vi "Process Live Data Q EMG.vi"(8 "error in (no error)":errorcluster, 10 "Live Data Q Elements":cluster{"NI Data Waveforms":waveform(dbl)[]}[](array[cluster]), 11 "NI Force Task in":refnum<class "NI Force Task.lvclass">) -> (0 "error out":errorcluster, 3 "NI Force Task out":refnum<class "NI Force Task.lvclass">)   [LabVIEW 2020, in "NI Force Task.lvlib" / "NI Force Task.lvclass"]
uses:
  NI Force Task.lvclass
  NI Force Task.lvclass/NI Force Task.ctl
  <vilib>/Analysis/baseanly.llb/Mean (DBL).vi
  <vilib>/Analysis/NI_AALBase.lvlib
  Task Viewer Messages/Receive Q Msg/Receive Q Msg.lvclass
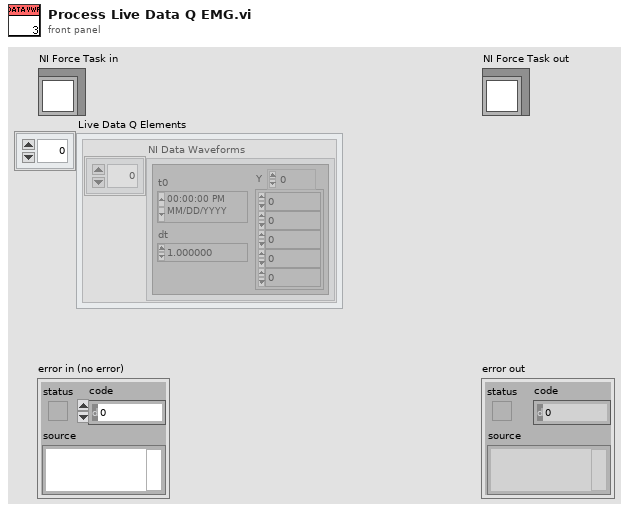
[diagram p1: front panel]
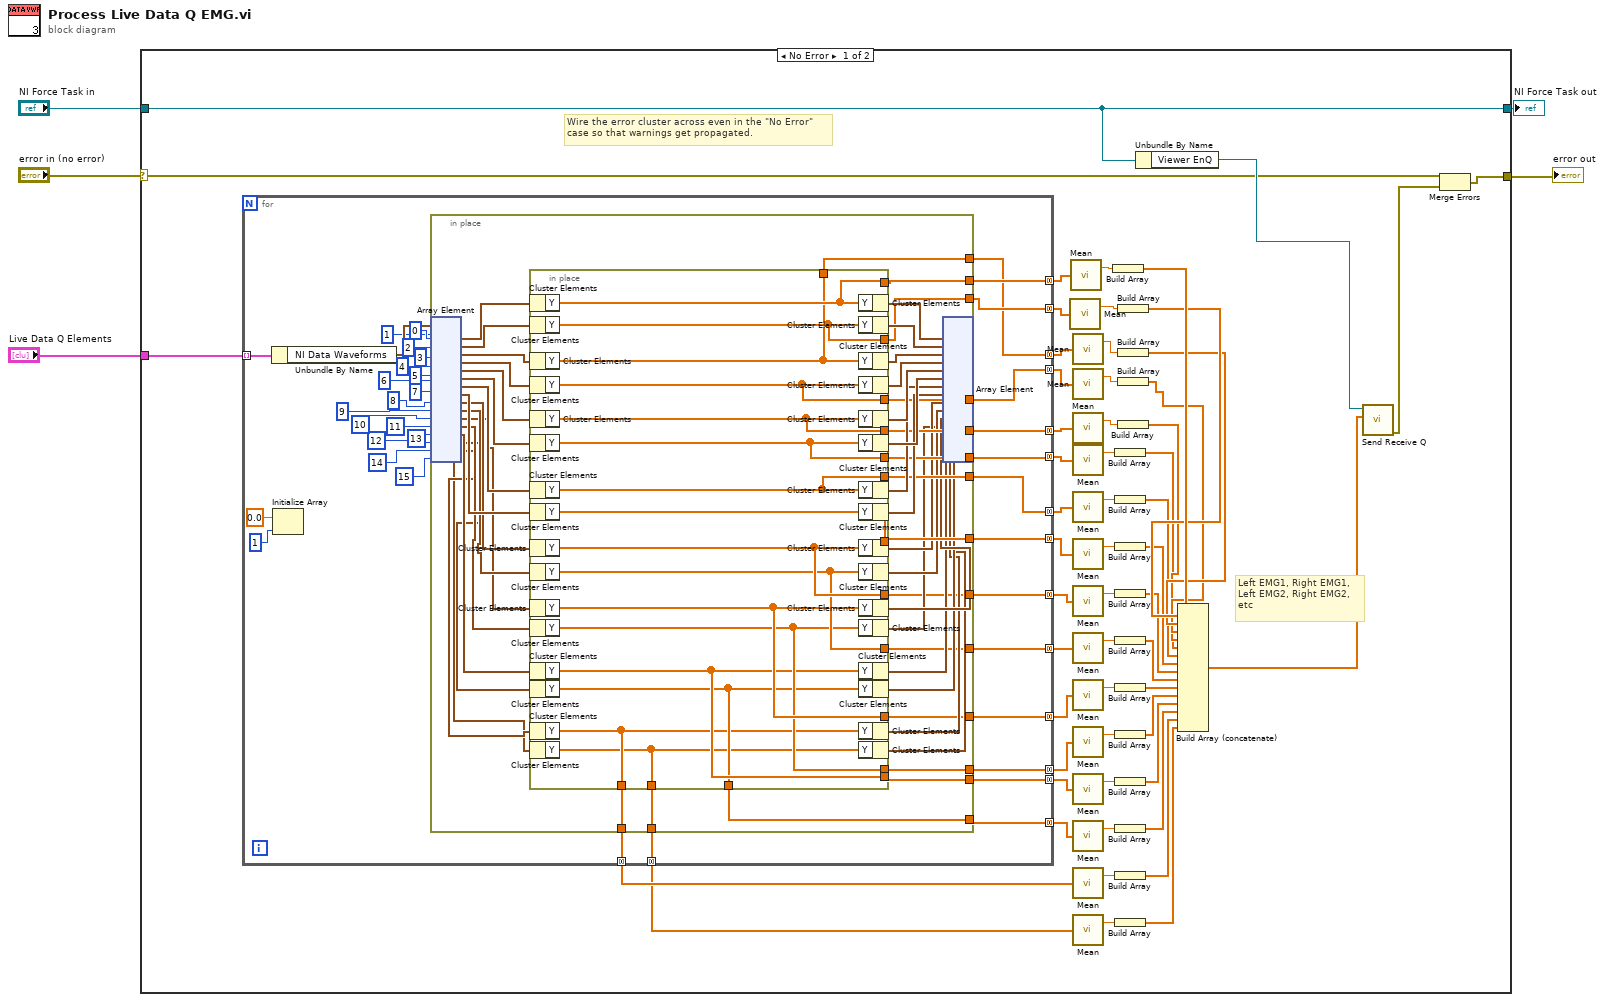
[diagram p0: block diagram]
diagram:
  n1 = case shown="No Error" "error in (no error)" {
    selector: "error in (no error)" -> [w53 w161]
    tunnel: [w60 w162] -> w3
    tunnel: "NI Force Task in" -> [w60 w162]
    tunnel: "Live Data Q Elements" -> [w59 _]
    tunnel: [w57 w161] -> w1
    frame No Error {
      # "Left EMG1, Right EMG1,\nLeft EMG2, Right EMG2,\netc"
      # "Wire the error cluster across even in the \"No Error\"\ncase so that warnings get propagated."
      n2 = for {
        tunnel: w59 -> [w96] mode=indexing
        tunnel: [w84] -> w52 mode=concatenating
        tunnel: [w83] -> w51 mode=concatenating
        tunnel: [w82] -> w48 mode=concatenating
        tunnel: [w81] -> w50 mode=concatenating
        tunnel: [w80] -> w49 mode=concatenating
        tunnel: [w79] -> w47 mode=concatenating
        tunnel: [w78] -> w46 mode=concatenating
        tunnel: [w77] -> w45 mode=concatenating
        tunnel: [w68] -> w13 mode=concatenating
        tunnel: [w67] -> w12 mode=concatenating
        tunnel: [w66] -> w11 mode=concatenating
        tunnel: [w65] -> w10 mode=concatenating
        tunnel: [w64] -> w9 mode=concatenating
        tunnel: [w63] -> w8 mode=concatenating
        tunnel: [w62] -> w7 mode=concatenating
        tunnel: [w61] -> w6 mode=concatenating
        n3 = Unbundle By Name(w96) -> ("NI Data Waveforms"=w93:waveform(dbl)[])
        n4 = Initialize Array(0.0 ("element"), 1 ("dimension size")) -> ()  [unwired: 1 out]
        n5 = in-place {
          in-place-border: [w128] -> w84
          in-place-border: [w127] -> w83
          in-place-border: [w126] -> w82
          in-place-border: [w125] -> w81
          in-place-border: [w124] -> w80
          in-place-border: [w123] -> w79
          in-place-border: [w122] -> w78
          in-place-border: [w121] -> w77
          in-place-border: [w104] -> w68
          in-place-border: [w103] -> w67
          in-place-border: [w102] -> w66
          in-place-border: [w101] -> w65
          in-place-border: [w100] -> w64
          in-place-border: [w99] -> w63
          in-place-border: [w98] -> w62
          in-place-border: [w97] -> w61
          n6 = in-place-array #1(w93, 0, 1, 2, 3, 4, 5, 6, 7, 8, 9, 10, 11, 12, 13, 14, 15) -> (w144:waveform(dbl), w143:waveform(dbl), w142:waveform(dbl), w141:waveform(dbl), w140:waveform(dbl), w139:waveform(dbl), w138:waveform(dbl), w137:waveform(dbl), w120:waveform(dbl), w119:waveform(dbl), w118:waveform(dbl), w117:waveform(dbl), w116:waveform(dbl), w115:waveform(dbl), w114:waveform(dbl), w113:waveform(dbl))
          n7 = in-place {
            in-place-border: [w160] -> w128
            in-place-border: [w159] -> w127
            in-place-border: [w158] -> w126
            in-place-border: [w157] -> w125
            in-place-border: [w156] -> w124
            in-place-border: [w155] -> w123
            in-place-border: [w154] -> w122
            in-place-border: [w153] -> w121
            in-place-border: [w152] -> w104
            in-place-border: [w151] -> w103
            in-place-border: [w150] -> w102
            in-place-border: [w149] -> w101
            in-place-border: [w148] -> w100
            in-place-border: [w147] -> w99
            in-place-border: [w146] -> w98
            in-place-border: [w145] -> w97
            n8 = in-place-cluster #2(w144) -> ("Y"=w160:dbl[])
            n9 = in-place-cluster #3(w143) -> ("Y"=w159:dbl[])
            n10 = in-place-cluster #4(w142) -> ("Y"=w158:dbl[])
            n11 = in-place-cluster #5(w141) -> ("Y"=w157:dbl[])
            n12 = in-place-cluster #6(w140) -> ("Y"=w156:dbl[])
            n13 = in-place-cluster #7(w139) -> ("Y"=w155:dbl[])
            n14 = in-place-cluster #8(w138) -> ("Y"=w154:dbl[])
            n15 = in-place-cluster #9(w137) -> ("Y"=w153:dbl[])
            n16 = in-place-cluster #10(w120) -> ("Y"=w152:dbl[])
            n17 = in-place-cluster #11(w119) -> ("Y"=w151:dbl[])
            n18 = in-place-cluster #12(w118) -> ("Y"=w150:dbl[])
            n19 = in-place-cluster #13(w117) -> ("Y"=w149:dbl[])
            n20 = in-place-cluster #14(w116) -> ("Y"=w148:dbl[])
            n21 = in-place-cluster #15(w115) -> ("Y"=w147:dbl[])
            n22 = in-place-cluster #16(w114) -> ("Y"=w146:dbl[])
            n23 = in-place-cluster #17(w113) -> ("Y"=w145:dbl[])
            n24 = in-place-cluster #2("Y"=w160) -> (w136:waveform(dbl))
            n25 = in-place-cluster #3("Y"=w159) -> (w135:waveform(dbl))
            n26 = in-place-cluster #4("Y"=w158) -> (w134:waveform(dbl))
            n27 = in-place-cluster #5("Y"=w157) -> (w133:waveform(dbl))
            n28 = in-place-cluster #6("Y"=w156) -> (w132:waveform(dbl))
            n29 = in-place-cluster #7("Y"=w155) -> (w131:waveform(dbl))
            n30 = in-place-cluster #8("Y"=w154) -> (w130:waveform(dbl))
            n31 = in-place-cluster #9("Y"=w153) -> (w129:waveform(dbl))
            n32 = in-place-cluster #10("Y"=w152) -> (w112:waveform(dbl))
            n33 = in-place-cluster #11("Y"=w151) -> (w111:waveform(dbl))
            n34 = in-place-cluster #12("Y"=w150) -> (w110:waveform(dbl))
            n35 = in-place-cluster #13("Y"=w149) -> (w109:waveform(dbl))
            n36 = in-place-cluster #14("Y"=w148) -> (w108:waveform(dbl))
            n37 = in-place-cluster #15("Y"=w147) -> (w107:waveform(dbl))
            n38 = in-place-cluster #16("Y"=w146) -> (w106:waveform(dbl))
            n39 = in-place-cluster #17("Y"=w145) -> (w105:waveform(dbl))
          }
          n40 = in-place-array #1(w136, w135, w134, w133, w132, w131, w130, w129, w112, w111, w110, w109, w108, w107, w106, w105) -> ()  [unwired: 17 out]
        }
      }
      n41 = call-poly <vilib>:"Mean.vi"("X"=w51) -> ("mean"=w54:dbl)  [unwired: 1 out]
      n42 = call-poly <vilib>:"Mean.vi"("X"=w52) -> ("mean"=w55:dbl)  [unwired: 1 out]
      n43 = call-poly <vilib>:"Mean.vi"("X"=w48) -> ("mean"=w44:dbl)  [unwired: 1 out]
      n44 = call-poly <vilib>:"Mean.vi"("X"=w50) -> ("mean"=w43:dbl)  [unwired: 1 out]
      n45 = call-poly <vilib>:"Mean.vi"("X"=w49) -> ("mean"=w42:dbl)  [unwired: 1 out]
      n46 = call-poly <vilib>:"Mean.vi"("X"=w47) -> ("mean"=w41:dbl)  [unwired: 1 out]
      n47 = call-poly <vilib>:"Mean.vi"("X"=w46) -> ("mean"=w40:dbl)  [unwired: 1 out]
      n48 = call-poly <vilib>:"Mean.vi"("X"=w45) -> ("mean"=w39:dbl)  [unwired: 1 out]
      n49 = call-poly <vilib>:"Mean.vi"("X"=w13) -> ("mean"=w29:dbl)  [unwired: 1 out]
      n50 = call-poly <vilib>:"Mean.vi"("X"=w12) -> ("mean"=w28:dbl)  [unwired: 1 out]
      n51 = call-poly <vilib>:"Mean.vi"("X"=w11) -> ("mean"=w27:dbl)  [unwired: 1 out]
      n52 = call-poly <vilib>:"Mean.vi"("X"=w10) -> ("mean"=w26:dbl)  [unwired: 1 out]
      n53 = call-poly <vilib>:"Mean.vi"("X"=w9) -> ("mean"=w25:dbl)  [unwired: 1 out]
      n54 = call-poly <vilib>:"Mean.vi"("X"=w8) -> ("mean"=w24:dbl)  [unwired: 1 out]
      n55 = call-poly <vilib>:"Mean.vi"("X"=w7) -> ("mean"=w23:dbl)  [unwired: 1 out]
      n56 = call-poly <vilib>:"Mean.vi"("X"=w6) -> ("mean"=w22:dbl)  [unwired: 1 out]
      n57 = Build Array(w55) -> (w37:dbl[])
      n58 = Build Array(w41) -> (w32:dbl[])
      n59 = Build Array(w40) -> (w31:dbl[])
      n60 = Build Array(w39) -> (w30:dbl[])
      n61 = Build Array(w29) -> (w21:dbl[])
      n62 = Build Array(w28) -> (w20:dbl[])
      n63 = Build Array(w27) -> (w19:dbl[])
      n64 = Build Array(w26) -> (w18:dbl[])
      n65 = Build Array(w25) -> (w17:dbl[])
      n66 = Build Array(w24) -> (w16:dbl[])
      n67 = Build Array(w23) -> (w15:dbl[])
      n68 = Build Array(w22) -> (w14:dbl[])
      n69 = Build Array(w54) -> (w36:dbl[])
      n70 = Build Array(w44) -> (w35:dbl[])
      n71 = Build Array(w43) -> (w34:dbl[])
      n72 = Build Array(w42) -> (w33:dbl[])
      n73 = Unbundle By Name(w60) -> ("Viewer EnQ"=w58:refnum<class "Message Enqueuer.lvclass">)
      n74 = Build Array (concatenate)(w37, w36, w35, w34, w33, w32, w31, w30, w21, w20, w19, w18, w17, w16, w15, w14) -> (w38:dbl[])
      n75 = call "Send Receive Q.vi"("Disp Data"=w38, "Message Enqueuer in"=w58) -> ("error out"=w56:errorcluster)  [unwired: 8 in, 1 out]
      n76 = Merge Errors(w53, w56) -> (w57:errorcluster)
    }
    frame Error {
    }
  }
  "error out" <- w1
  "NI Force Task out" <- w3
